vi "write_new_Flash.vi"(0 "address (3 bytes)":u32, 1 "sector erase":bool, 2 "write array":u8[](array[numeric]) format="%x") -> ()   [LabVIEW 2022 SP3]
panel:
  in  "address (3 bytes) 2":u32
  out "InputReport1":u8[](array[numeric]) format="%x"
  out "Output Report":u8[](array[numeric])
  out "Input Report":u8[](array[numeric])
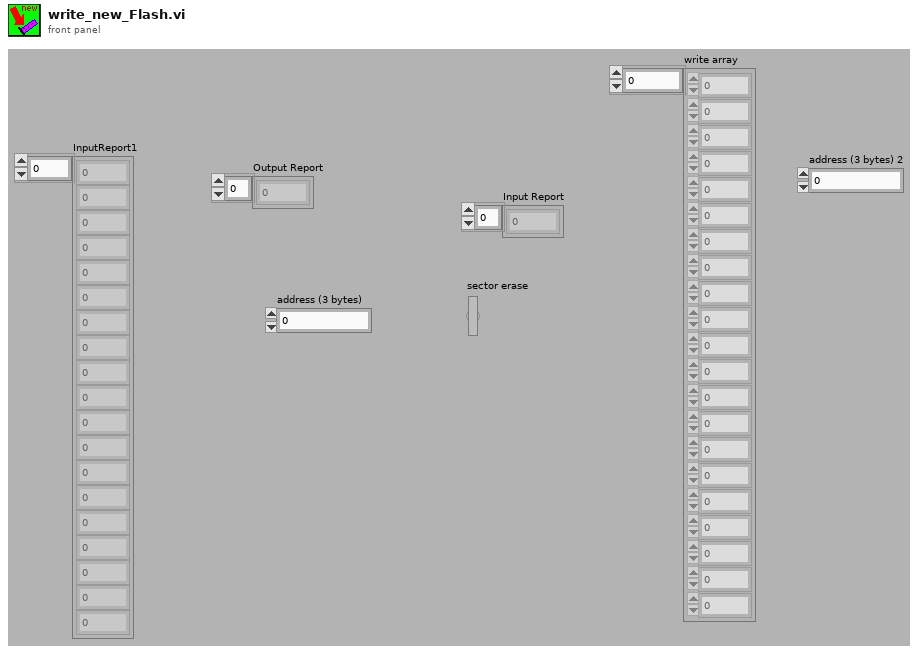
[diagram p1: front panel]
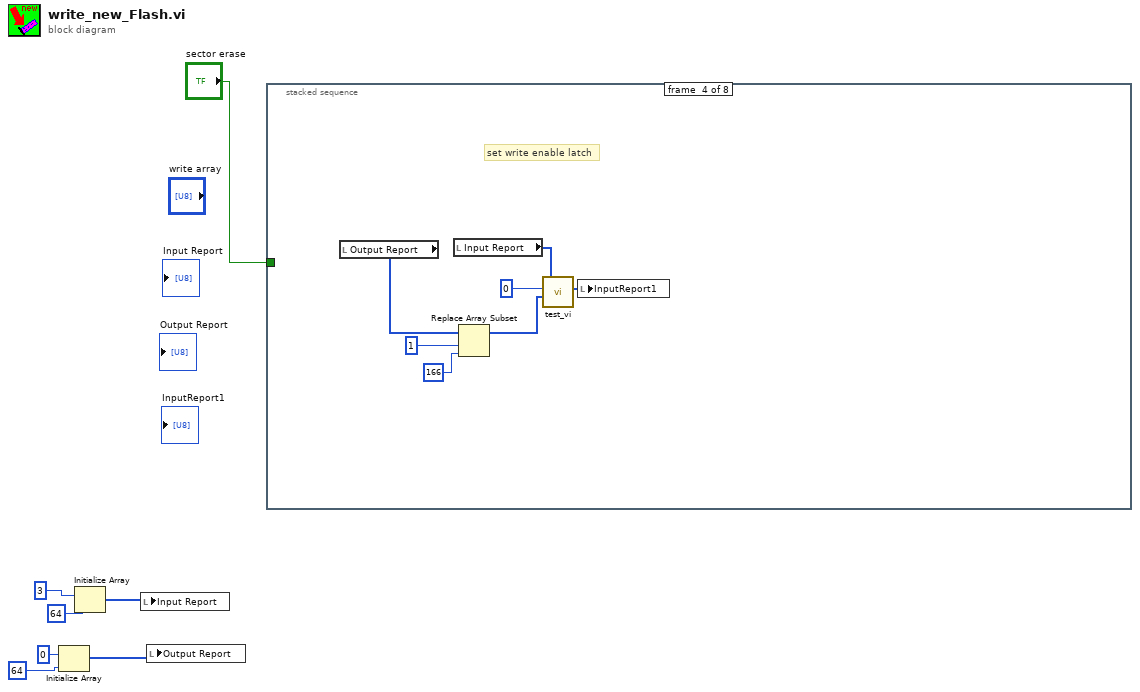
[diagram p0: block diagram]
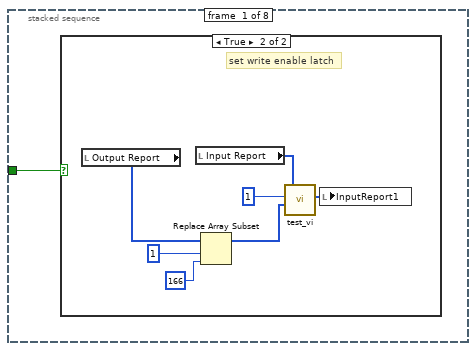
[diagram p2: hidden frame]
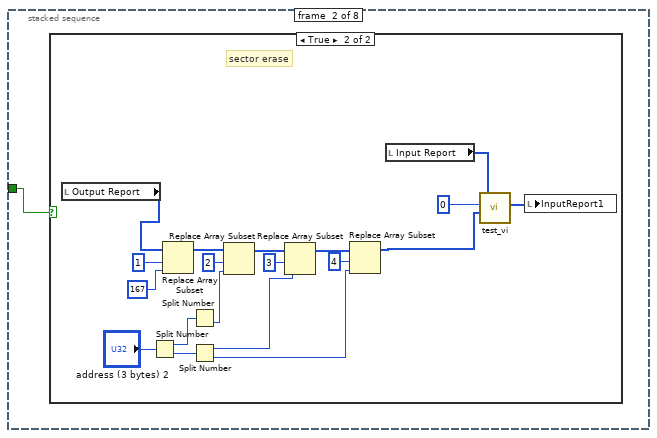
[diagram p4: hidden frame]
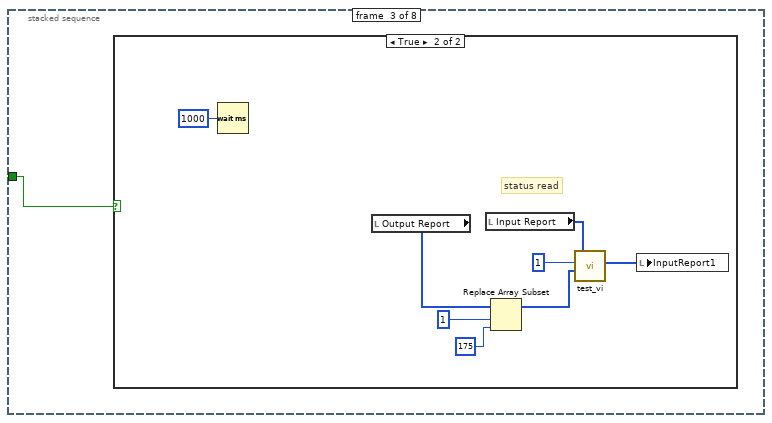
[diagram p6: hidden frame]
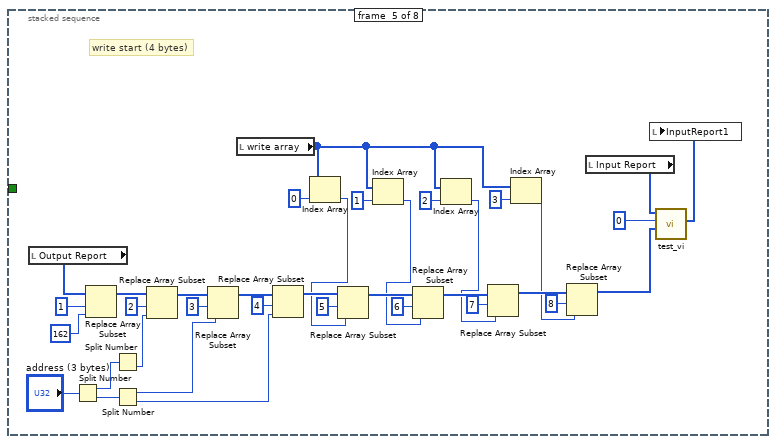
[diagram p8: hidden frame]
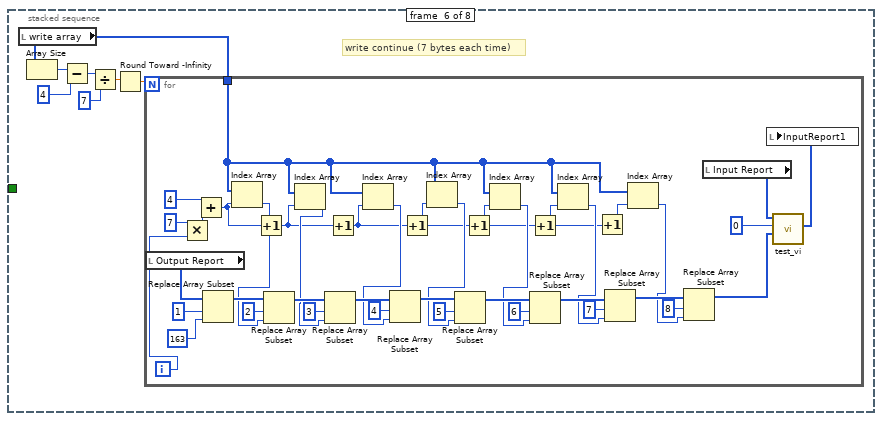
[diagram p9: hidden frame]
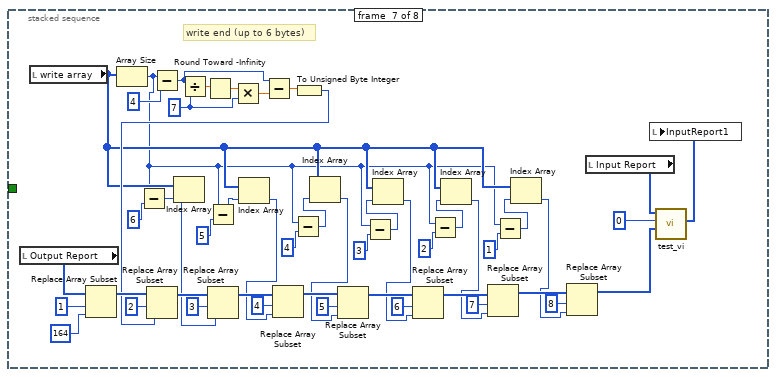
[diagram p10: hidden frame]
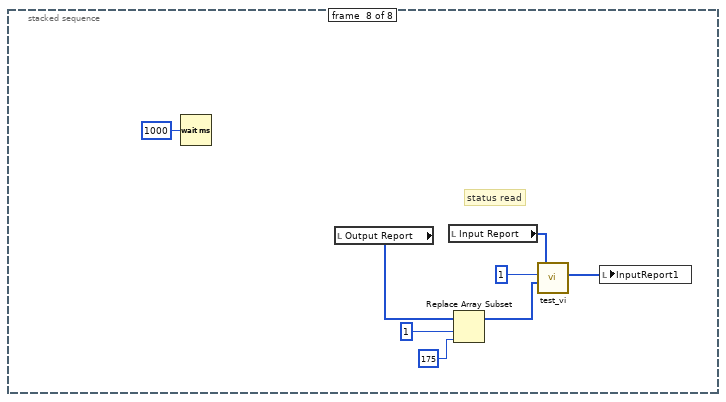
[diagram p11: hidden frame]
diagram:
  n1 = Initialize Array(u8 0 ("element"), 64 ("dimension size")) -> (w2:u8[])
  n2 = Initialize Array(u8 3 ("element"), 64 ("dimension size")) -> (w3:u8[])
  n3 = local write "Input Report"(w3) -> ()
  n4 = local write "Output Report"(w2) -> ()
  n5 = stacked-sequence {
    tunnel: "sector erase" -> [w8 w16 w36 _ _ _ _ _]
    frame #0 {
      n6 = case shown="True" w8 {
        frame False {
        }
        frame True {
          # "set write enable latch"
          n7 = local read "Output Report"() -> (w12:u8[])
          n8 = local read "Input Report"() -> (w11:u8[])
          n9 = Replace Array Subset(array=w12, new element=u8 166 ("new element/subarray"), index=1) -> (w10:u8[])
          n10 = call "test_vi.vi"("OutputReport_in"=w10, "DevDet_in"=1, "InputReport_in"=w11) -> ("InputReport_out"=w9:u8[])  [unwired: 1 in, 3 out]
          n11 = local write "InputReport1"(w9) -> ()
        }
      }
    }
    frame #1 {
      n12 = case shown="True" w16 {
        frame False {
        }
        frame True {
          # "sector erase"
          n13 = local read "Output Report"() -> (w19:u8[])
          n14 = Split Number(x="address (3 bytes) 2") -> (hi(x)=w32:u16, lo(x)=w31:u16)
          n15 = Replace Array Subset(array=w19, new element=u8 167 ("new element/subarray"), index=1) -> (w30:u8[])
          n16 = Split Number(x=w32) -> (lo(x)=w29:u8)  [unwired: 1 out]
          n17 = Split Number(x=w31) -> (hi(x)=w26:u8, lo(x)=w23:u8)
          n18 = Replace Array Subset(array=w30, new element=w29, index=2) -> (w27:u8[])
          n19 = Replace Array Subset(array=w27, new element=w26, index=3) -> (w24:u8[])
          n20 = Replace Array Subset(array=w24, new element=w23, index=4) -> (w20:u8[])
          n21 = local read "Input Report"() -> (w18:u8[])
          n22 = call "test_vi.vi"("OutputReport_in"=w20, "DevDet_in"=0, "InputReport_in"=w18) -> ("InputReport_out"=w17:u8[])  [unwired: 1 in, 3 out]
          n23 = local write "InputReport1"(w17) -> ()
        }
      }
    }
    frame #2 {
      n24 = case shown="True" w36 {
        frame False {
        }
        frame True {
          # "status read"
          n25 = Wait (ms)(milliseconds to wait=u32 1000) -> ()  [unwired: 1 out]
          n26 = local read "Output Report"() -> (w40:u8[])
          n27 = local read "Input Report"() -> (w39:u8[])
          n28 = Replace Array Subset(array=w40, new element=u8 175 ("new element/subarray"), index=1) -> (w38:u8[])
          n29 = call "test_vi.vi"("OutputReport_in"=w38, "DevDet_in"=1, "InputReport_in"=w39) -> ("InputReport_out"=w37:u8[])  [unwired: 1 in, 3 out]
          n30 = local write "InputReport1"(w37) -> ()
        }
      }
    }
    frame #3 {
      # "set write enable latch"
      n31 = local read "Output Report"() -> (w48:u8[])
      n32 = local read "Input Report"() -> (w47:u8[])
      n33 = Replace Array Subset(array=w48, new element=u8 166 ("new element/subarray"), index=1) -> (w46:u8[])
      n34 = call "test_vi.vi"("OutputReport_in"=w46, "DevDet_in"=0, "InputReport_in"=w47) -> ("InputReport_out"=w45:u8[])  [unwired: 1 in, 3 out]
      n35 = local write "InputReport1"(w45) -> ()
    }
    frame #4 {
      # "write start (4 bytes)"
      n36 = local read "Output Report"() -> (w84:u8[])
      n37 = Split Number(x="address (3 bytes)") -> (hi(x)=w80:u16, lo(x)=w79:u16)
      n38 = Replace Array Subset(array=w84, new element=u8 162 ("new element/subarray"), index=1) -> (w78:u8[])
      n39 = Split Number(x=w80) -> (lo(x)=w77:u8)  [unwired: 1 out]
      n40 = Split Number(x=w79) -> (hi(x)=w74:u8, lo(x)=w71:u8)
      n41 = Replace Array Subset(array=w78, new element=w77, index=2) -> (w75:u8[])
      n42 = Replace Array Subset(array=w75, new element=w74, index=3) -> (w72:u8[])
      n43 = local read "write array"() -> (w60:u8[])
      n44 = Replace Array Subset(array=w72, new element=w71, index=4) -> (w69:u8[])
      n45 = Index Array(array=w60, index=0) -> (element=w55:u8)
      n46 = Replace Array Subset(array=w69, new element=w55, index=5) -> (w68:u8[])
      n47 = Index Array(array=w60, index=1) -> (element=w54:u8)
      n48 = Replace Array Subset(array=w68, new element=w54, index=6) -> (w67:u8[])
      n49 = Index Array(array=w60, index=2) -> (element=w53:u8)
      n50 = Replace Array Subset(array=w67, new element=w53, index=7) -> (w66:u8[])
      n51 = Index Array(array=w60, index=3) -> (element=w52:u8)
      n52 = Replace Array Subset(array=w66, new element=w52, index=8) -> (w65:u8[])
      n53 = local read "Input Report"() -> (w83:u8[])
      n54 = call "test_vi.vi"("OutputReport_in"=w65, "DevDet_in"=0, "InputReport_in"=w83) -> ("InputReport_out"=w82:u8[])  [unwired: 1 in, 3 out]
      n55 = local write "InputReport1"(w82) -> ()
    }
    frame #5 {
      # "write continue (7 bytes each time)"
      n56 = local read "write array"() -> (w88:u8[])
      n57 = Array Size(array=w88) -> (size(s)=w94:i32)
      n58 = Subtract(x=w94, y=4) -> (x-y=w92:i32)
      n59 = Divide(x=w92, y=7) -> (x/y=w90:dbl)
      n60 = Round Toward -Infinity(1:w90) -> (0:w89:dbl)
      n61 = for {
        N: w89 -> [_]
        tunnel: w88 -> [w106]
        i -> [w105]
        n62 = local read "Output Report"() -> (w131:u8[])
        n63 = Multiply(x=7, y=w105) -> (x*y=w103:i32)
        n64 = Add(x=4, y=w103) -> (x+y=w101:i32)
        n65 = Replace Array Subset(array=w131, new element=u8 163 ("new element/subarray"), index=1) -> (w128:u8[])
        n66 = Index Array(array=w106, index=w101) -> (element=w107:u8)
        n67 = Increment(x=w101) -> (x+1=w100:i32)
        n68 = Replace Array Subset(array=w128, new element=w107, index=2) -> (w126:u8[])
        n69 = Index Array(array=w106, index=w100) -> (element=w108:u8)
        n70 = Replace Array Subset(array=w126, new element=w108, index=3) -> (w124:u8[])
        n71 = Increment(x=w100) -> (x+1=w99:i32)
        n72 = Index Array(array=w106, index=w99) -> (element=w109:u8)
        n73 = Replace Array Subset(array=w124, new element=w109, index=4) -> (w122:u8[])
        n74 = Increment(x=w99) -> (x+1=w98:i32)
        n75 = Index Array(array=w106, index=w98) -> (element=w113:u8)
        n76 = Replace Array Subset(array=w122, new element=w113, index=5) -> (w121:u8[])
        n77 = Increment(x=w98) -> (x+1=w97:i32)
        n78 = Index Array(array=w106, index=w97) -> (element=w112:u8)
        n79 = Increment(x=w97) -> (x+1=w95:i32)
        n80 = Replace Array Subset(array=w121, new element=w112, index=6) -> (w120:u8[])
        n81 = Index Array(array=w106, index=w95) -> (element=w111:u8)
        n82 = Increment(x=w95) -> (x+1=w96:i32)
        n83 = Replace Array Subset(array=w120, new element=w111, index=7) -> (w119:u8[])
        n84 = Index Array(array=w106, index=w96) -> (element=w110:u8)
        n85 = Replace Array Subset(array=w119, new element=w110, index=8) -> (w118:u8[])
        n86 = local read "Input Report"() -> (w130:u8[])
        n87 = call "test_vi.vi"("OutputReport_in"=w118, "DevDet_in"=0, "InputReport_in"=w130) -> ("InputReport_out"=w129:u8[])  [unwired: 1 in, 3 out]
        n88 = local write "InputReport1"(w129) -> ()
      }
    }
    frame #6 {
      w155 = 7 ("y")
      # "write end (up to 6 bytes)"
      n89 = local read "Output Report"() -> (w180:u8[])
      n90 = local read "write array"() -> (w150:u8[])
      n91 = Replace Array Subset(array=w180, new element=u8 164 ("new element/subarray"), index=1) -> (w177:u8[])
      n92 = Array Size(array=w150) -> (size(s)=w135:i32)
      n93 = Subtract(x=w135, y=6) -> (x-y=w147:i32)
      n94 = Subtract(x=w135, y=4) -> (x-y=w153:i32)
      n95 = Index Array(array=w150, index=w147) -> (element=w148:u8)
      n96 = Divide(x=w153, y=w155) -> (x/y=w157:dbl)
      n97 = Round Toward -Infinity(1:w157) -> (0:w156:dbl)
      n98 = Subtract(x=w135, y=5) -> (x-y=w144:i32)
      n99 = Multiply(x=w156, y=w155) -> (x*y=w154:dbl)
      n100 = Index Array(array=w150, index=w144) -> (element=w149:u8)
      n101 = Subtract(x=w153, y=w154) -> (x-y=w152:dbl)
      n102 = Subtract(x=w135, y=4) -> (x-y=w142:i32)
      n103 = To Unsigned Byte Integer(number=w152) -> (unsigned 8bit integer=w151:u8)
      n104 = Replace Array Subset(array=w177, new element=w151, index=2) -> (w175:u8[])
      n105 = Replace Array Subset(array=w175, new element=w148, index=3) -> (w173:u8[])
      n106 = Replace Array Subset(array=w173, new element=w149, index=4) -> (w171:u8[])
      n107 = Index Array(array=w150, index=w142) -> (element=w162:u8)
      n108 = Replace Array Subset(array=w171, new element=w162, index=5) -> (w170:u8[])
      n109 = Subtract(x=w135, y=3) -> (x-y=w140:i32)
      n110 = Index Array(array=w150, index=w140) -> (element=w161:u8)
      n111 = Replace Array Subset(array=w170, new element=w161, index=6) -> (w169:u8[])
      n112 = Subtract(x=w135, y=2) -> (x-y=w138:i32)
      n113 = Index Array(array=w150, index=w138) -> (element=w160:u8)
      n114 = Replace Array Subset(array=w169, new element=w160, index=7) -> (w168:u8[])
      n115 = Subtract(x=w135, y=1) -> (x-y=w136:i32)
      n116 = Index Array(array=w150, index=w136) -> (element=w159:u8)
      n117 = Replace Array Subset(array=w168, new element=w159, index=8) -> (w167:u8[])
      n118 = local read "Input Report"() -> (w179:u8[])
      n119 = call "test_vi.vi"("OutputReport_in"=w167, "DevDet_in"=0, "InputReport_in"=w179) -> ("InputReport_out"=w178:u8[])  [unwired: 1 in, 3 out]
      n120 = local write "InputReport1"(w178) -> ()
    }
    frame #7 {
      # "status read"
      n121 = Wait (ms)(milliseconds to wait=u32 1000) -> ()  [unwired: 1 out]
      n122 = local read "Output Report"() -> (w187:u8[])
      n123 = local read "Input Report"() -> (w186:u8[])
      n124 = Replace Array Subset(array=w187, new element=u8 175 ("new element/subarray"), index=1) -> (w185:u8[])
      n125 = call "test_vi.vi"("OutputReport_in"=w185, "DevDet_in"=1, "InputReport_in"=w186) -> ("InputReport_out"=w184:u8[])  [unwired: 1 in, 3 out]
      n126 = local write "InputReport1"(w184) -> ()
    }
  }
